vi "_GetConfigPath.vi"(8 "error in (no error)":errorcluster, 10 "file path(empty for default) in":path, 11 "DB Ref":T1) -> (0 "error out":errorcluster, 2 "file path(empty for default) out":path, 3 "DB Ref(dup)":T1)   [LabVIEW 2014, in "TagDB(dev).lvlib"]
uses:
  TagDB(dev).lvlib
  tagDB_Def.ctl
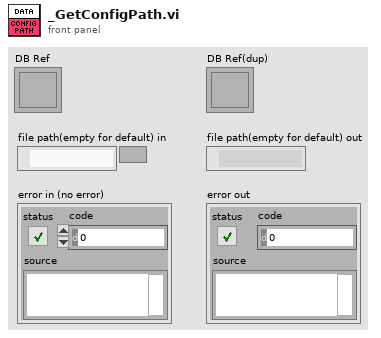
[diagram p1: front panel]
types:
  T1 = typedef "TagDB(dev).lvlib/tagDB_Def.ctl" = refnum<k1>
  T2 = typedef "TagDB.lvlib/DEF-DATA.ctl" = cluster{"data hashmap":variant, "DataChangeFlag":i64, "ItemChangeFlag":i64, "name":string}
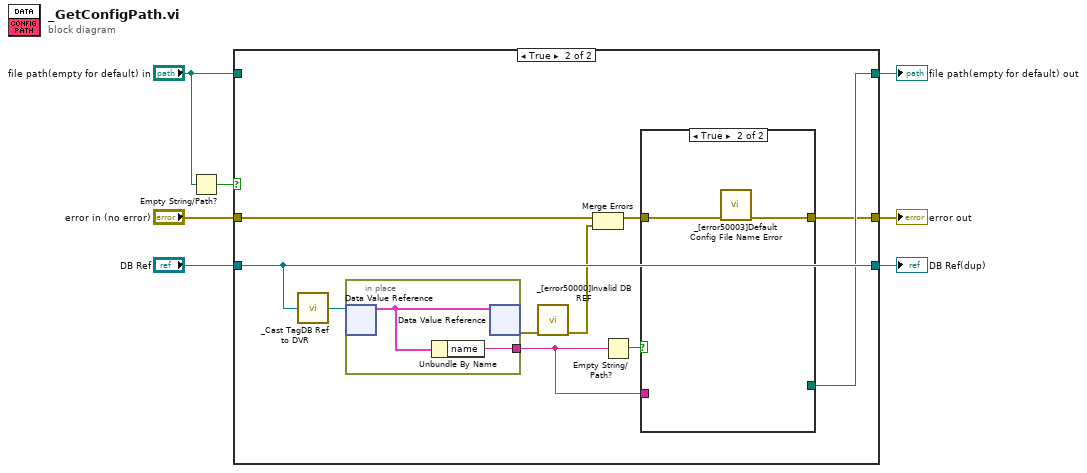
[diagram p0: block diagram]
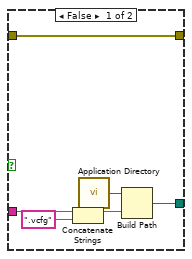
[diagram p3: hidden frame]
diagram:
  n1 = Empty String/Path?(string/path="file path(empty for default) in") -> (empty?=w1:bool)
  n2 = case shown="True" w1 {
    tunnel: "file path(empty for default) in" -> [w10 _]
    tunnel: [w10 w15] -> w3
    tunnel: [w9 w19] -> w4
    tunnel: "DB Ref" -> [w9 w19]
    tunnel: [w8 w14] -> w6
    tunnel: "error in (no error)" -> [w8 w13]
    frame False {
    }
    frame True {
      n3 = call "_Cast TagDB Ref to DVR.vi"("TagDB"=w19) -> ("DVR"=w20:refnum<data-value>)  [unwired: 4 in]
      n4 = in-place {
        in-place-border: [w29] -> w16
        n5 = in-place-dvr #1(w20) -> (w30:T2)  [unwired: 1 out]
        n6 = Unbundle By Name(w30) -> ("name"=w29:string)
        n7 = in-place-dvr #1(w30) -> (w18:errorcluster)  [unwired: 1 out]
      }
      n8 = call "_[error50000]Invalid DB REF.vi"("error in (no error)"=w18) -> ("error out"=w11:errorcluster)  [unwired: 10 in]
      n9 = Merge Errors(w13, w11) -> (w12:errorcluster)
      n10 = Empty String/Path?(string/path=w16) -> (empty?=w17:bool)
      n11 = case shown="True" w17 {
        tunnel: w16 -> [w25 _]
        tunnel: [w24 _] -> w15
        tunnel: [w23 w27] -> w14
        tunnel: w12 -> [w23 w28]
        frame False {
          n12 = Concatenate Strings(w25, ".vcfg" ("string")) -> (w22:string)
          n13 = call <vilib>:"Application Directory.vi"() -> ("Application Directory"=w26:path)
          n14 = Build Path(base path=w26, name or relative path=w22) -> (appended path=w24:path)
        }
        frame True {
          n15 = call "_[error50003]Default Config File Name Error.vi"("error in (no error)"=w28) -> ("error out"=w27:errorcluster)  [unwired: 10 in]
        }
      }
    }
  }
  "error out" <- w6
  "DB Ref(dup)" <- w4
  "file path(empty for default) out" <- w3
